vi "Vector_Normalization.vi"(8 "error in":errorcluster, 11 "Input vector":dbl[](array[numeric])) -> (0 "error out":errorcluster, 3 "Normalized vector":dbl[](array[numeric]))   [LabVIEW 2023]
doc: "This VI is used to normalize an input vector.\nIf an Inf value is detected, it is replaced by a NaN, ditto for -Inf values.\n\nHow it's done:\n1- Check the Inf or -Inf values\n2- Create a 1/0 vector from this vector of Bouléens (True becomes 0 and False becomes 0).\n3- Multiply the original vector by this 0/1 vector. Inf or -Inf values become NaN"
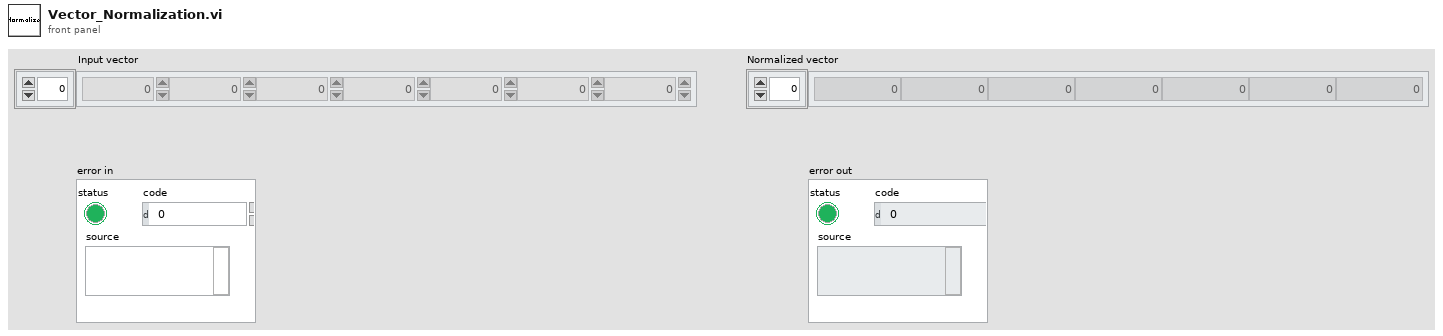
[diagram p1: front panel]
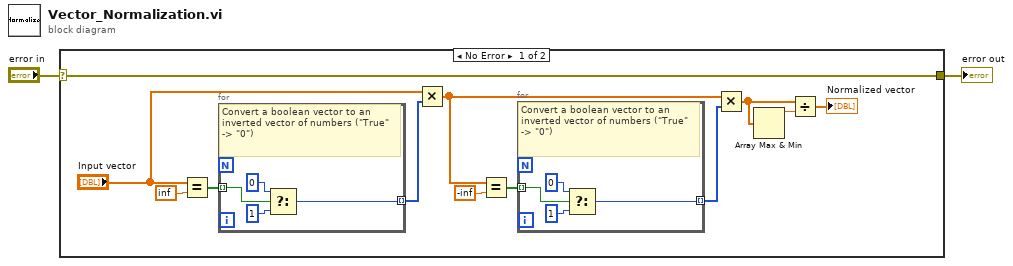
[diagram p0: block diagram]
diagram:
  n1 = case shown="No Error" "error in" {
    selector: "error in" -> [w14 w23]
    tunnel: [w14 w23] -> w1
    frame No Error {
      n2 = Equal?(x="Input vector", y=inf) -> (x = y?=w12:bool[])
      n3 = for {
        tunnel: w12 -> [w22] mode=indexing
        tunnel: [w19] -> w11 mode=indexing
        # "Convert a boolean vector to an inverted vector of numbers (\"True\" -> \"0\")"
        n4 = Select(t=u8 0, s=w22, f=u8 1 ("t")) -> (s? t:f=w19:u8)
      }
      n5 = Multiply(x="Input vector", y=w11) -> (x*y=w8:dbl[])
      n6 = Equal?(x=w8, y=-inf) -> (x = y?=w10:bool[])
      n7 = for {
        tunnel: w10 -> [w18] mode=indexing
        tunnel: [w15] -> w7 mode=indexing
        # "Convert a boolean vector to an inverted vector of numbers (\"True\" -> \"0\")"
        n8 = Select(t=u8 0, s=w18, f=u8 1 ("t")) -> (s? t:f=w15:u8)
      }
      n9 = Multiply(x=w8, y=w7) -> (x*y=w6:dbl[])
      n10 = Array Max & Min(array=w6) -> (max value=w5:dbl)  [unwired: 3 out]
      n11 = Divide(x=w6, y=w5) -> (x/y=→"Normalized vector":dbl[])
    }
    frame Error {
    }
  }
  "error out" <- w1
